vi "Multi-Device_Sync-AI_and_AO-Shared_Timebase_&_Trig-DSA SINGLE DEVICE.vi"() -> ()   [LabVIEW 2020]
doc: "I. Description:\nThis example configures a total of four tasks on two PXI Dynamic Signal Acquistion (DSA) devices. Each device runs a task for analog input and another for analog output. This VI illustrates continuous analog input and ouptut operations.\n\nII. Instructions for Running:\n1. Select which type of Syncrhonization method you want to use.\n2. Select the physical channels to corresponding to the signal connection on each device.\n3. Enter the minimum and maximum expected voltage for the input and output operations on each device.\nNote: For optimal accuracy, match the input range to the expected voltage level of the measured signal (for input) and generated signal (for output).\n4. Set the number of samples to acquire per channel. This parameter determines how many points will be read and generated with each iteration of the WHILE loop.\n5. Set the rate of the acquisition and generation. The same sampling rate is employed for input and output operations on each device.\nNote: The sampling rate should be at least 2.2 times the maximum frequency component of the signal being acquired on analog input and the signal being generated on analog output. Frequency components beyond about 0.47 times the sampling rate will be eliminated by the alias and imaging protection on the DSA device.\n\nIII. Block Diagram Steps:\n1. Create an analog input and output channel for both the master and slave devices.\n2. Set timing parameters for a continuous acquisition. The sample rate and block size are set to the same values for each device.\n3. There are two types of synchronization available on DSA devices. The first method shares the Sample Clock Timebase across the PXI_Star bus. It also uses the Sync Pulse which is shared across the PXI_Trig / RTSI bus. The second method uses the Sync Pulse in conjunction with the PXI Reference clock 10 on the PXI backplane. \n4. Call the Get Terminal Name with Device Prefix VI to append the device name to the signal name for the acquisition start trigger. This signal is then used as an output generation trigger on the master as well as and acquisition start trigger and generation start trigger on the slave. The signal is shared along the PXI_Trig / RTSI bus.\n5. Synthesize a standard waveform (sine, square, or triangle) and load this data into the output RAM buffer for each device.\n6. Call the Start VI to start the acquisition and generation tasks. (Note: The flat case structure provides flow control so that the slave device is armed before the master so that the slave device does not miss the trigger.)\n7. Read all of the waveform data from both devices.\n8. Check the status of the analog output tasks on both devices.\n9. Call the Clear Task VI to stop the acquisition and generation and clear the task.\n10. Use the popup dialog box to display an error if any.\n\nIV. I/O Connections Overview:\nMake sure your signal input and output terminals matches the Physical Channel I/O controls.\n\nIt is important to ensure that your PXI chassis has been properly configured in MAX. If your chassis has not been configured in software before running the VI, your devices may fail to synchronize properly."
uses:
  <vilib>/Utility/error.llb/DialogType.ctl
  <vilib>/DAQmx/write.llb/DAQmx Write (Analog Wfm 1Chan NSamp).vi
  <vilib>/DAQmx/create/channels.llb/DAQmx Create Channel (AI-Voltage-Basic).vi
  <vilib>/DAQmx/create/channels.llb/DAQmx Create Channel (AO-Voltage-Basic).vi
  <vilib>/DAQmx/configure/timing.llb/DAQmx Timing (Sample Clock).vi
  <vilib>/DAQmx/configure/trigger.llb/DAQmx Start Trigger (Digital Edge).vi
  <vilib>/DAQmx/miscellaneous.llb/DAQmx Fill In Error Info.vi
  <vilib>/DAQmx/read.llb/DAQmx Read (Analog 1D Wfm NChan NSamp).vi
  <resource>/objmgr/daqmx.rc
panel:
  out "Resulting Sample \nClock Rate [S/s]":dbl format="%.2f"
  in  "Desired Frequency":dbl=1000.0 format="%.2f"
  in  "Cycles per Buffer":dbl=5.0 format="%.2f"
  in  "Waveform Type":T1(ring)
  in  "Samples per Buffer":dbl=250.0
  in  "Amplitude":dbl=1.0 format="%0.2p"
  in  "Samples per Channel":i32=2000 caption="Samples to Read per Loop"
  in  "Minimum Value":dbl=-10.0 caption="Output Minimum Value" format="%0.2f"
  in  "Maximum Value":dbl=10.0 caption="Output Maximum Value" format="%0.2f"
  in  "Physical Channel":tag="PXI1Slot2/ao0" caption="Master Output Physical Channels"
  in  "Maximum Value":dbl=10.0 caption="Input Maximum Value" format="%0.2f"
  in  "Minimum Value":dbl=-10.0 caption="Input Minimum Value" format="%0.2f"
  in  "Physical Channel":tag="PXI1Slot2/ai0" caption="Master Input Physical Channel"
  in  "stop":bool
  out "Measurement":waveform(dbl)[](graph) caption="Measurement:  Master Board"
  # "For instructions, select Help>>Show Context Help"
  # "Channel Parameters:  Master Board"
  # "Timing Parameters"
  # "Waveform Information"
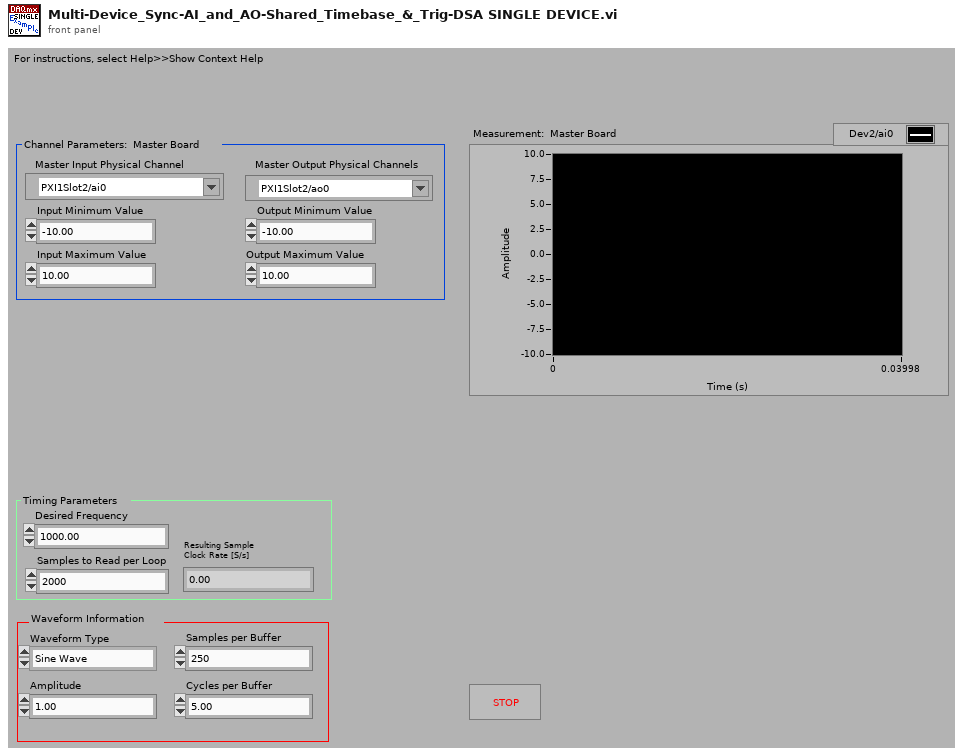
[diagram p1: front panel]
types:
  T1 = enum16{"Sine Wave", "Triangle Wave", "Square Wave", "Sawtooth Wave"}
  T2 = typedef "DialogType.ctl" = u16
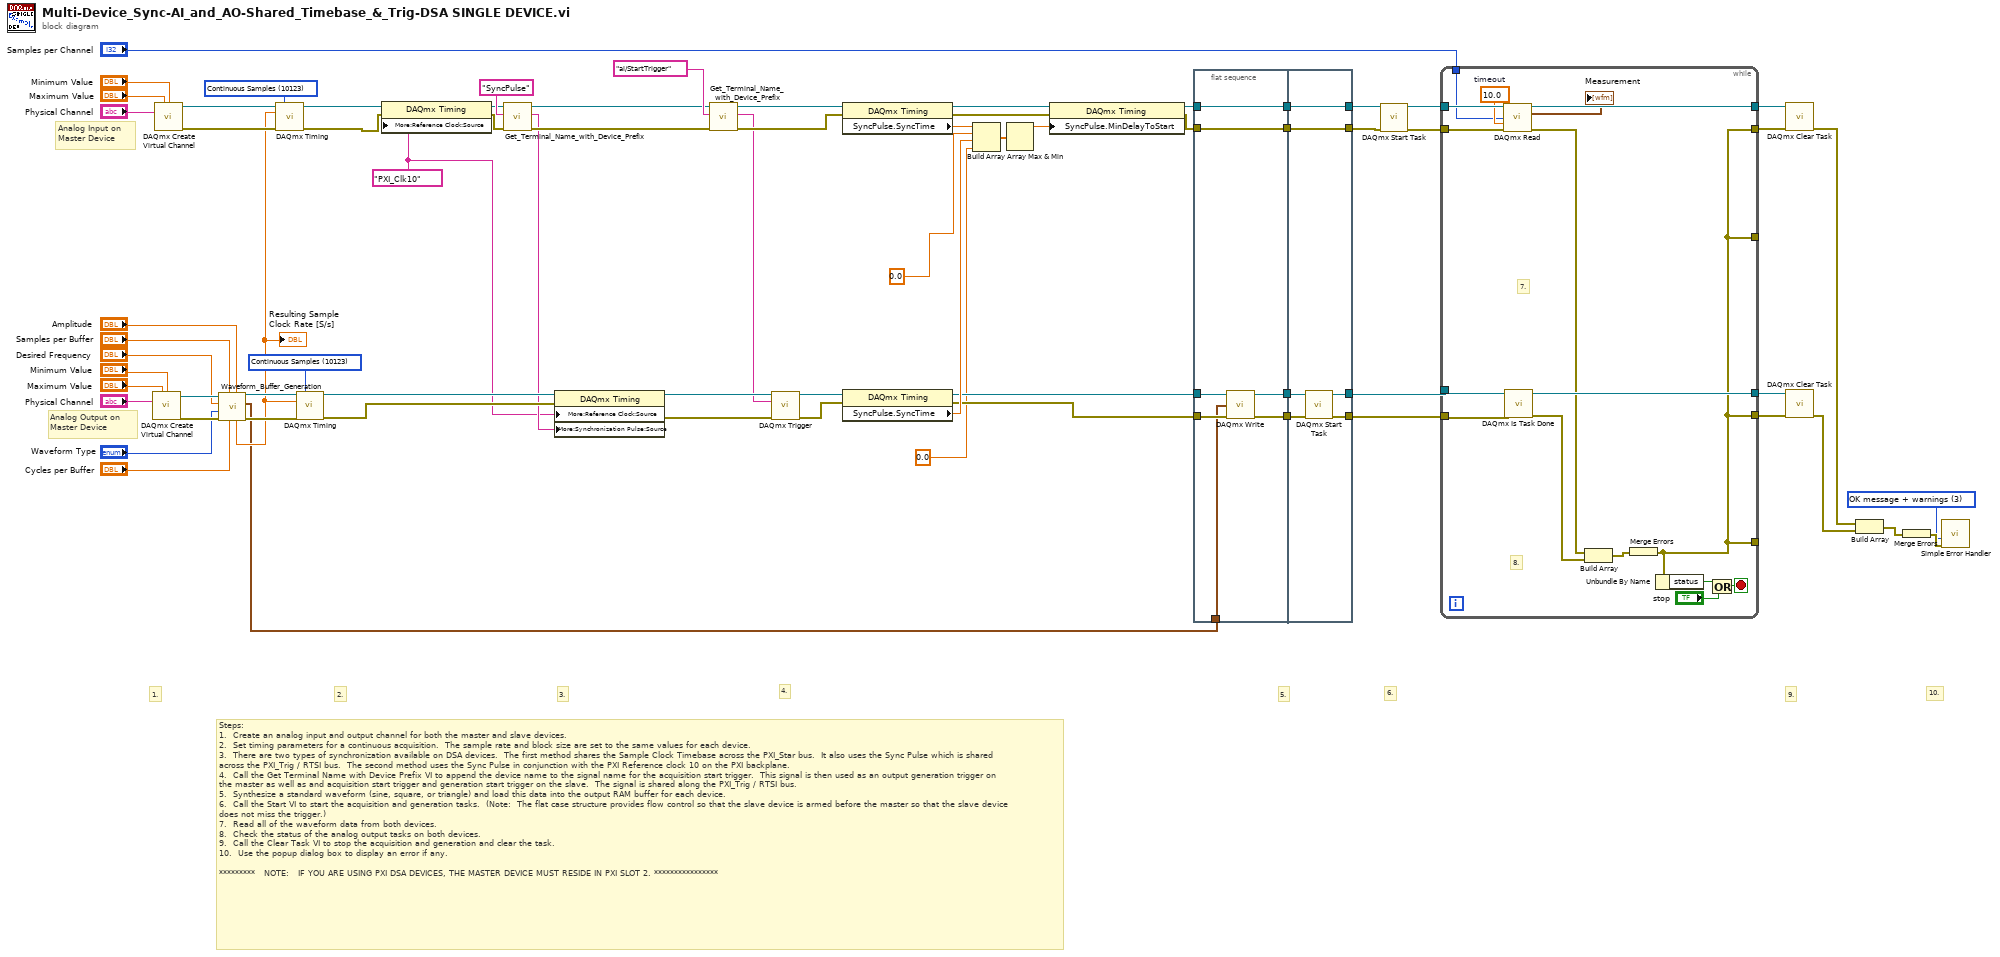
[diagram p0: block diagram]
diagram:
  w3 = tag "PXI_Clk10" ("RefClk.Src")
  w42 = T2 3 items=["no dialog", "OK message", "continue or stop message", "OK message + warnings", "continue/stop + warnings"] ("type of dialog (OK msg:1)")
  w65 = 10123 items=["Finite Samples"=10178, "Continuous Samples"=10123] ("sample mode")
  w68 = 10123 items=["Finite Samples"=10178, "Continuous Samples"=10123] ("sample mode")
  # "Analog Output on\nMaster Device"
  # "Analog Input on\nMaster Device"
  # "10."
  # "9."
  # "Steps: \n1.  Create an analog input and output channel for both the master and slave devices.\n2.  Set timing parameters for a continuous acquisition.  The sample rate and block size are set to the same values for each device.\n3.  There are two types of synchronization available on DSA devices.  The first method shares the Sample Clock Timebase across the PXI_Star bus.  It also uses the Sync Pulse which is shared across the PXI_Trig / RTSI bus.  The second method uses the Sync Pulse in conjunction with the PXI Reference clock 10 on the PXI backplane. \n4.  Call the Get Terminal Name with Device Prefix VI to append the device name to the signal name for the acquisition start trigger.  This signal is then used as an output generation trigger on the master as well as and acquisition start trigger and generation start trigger on the slave.  The signal is shared along the PXI_Trig / RTSI bus.\n5.  Synthesize a standard waveform (sine, square, or triangle) and load this data into the output RAM buffer for each device.\n6.  Call the Start VI to start the acquisition and generation tasks.  (Note:  The flat case structure provides flow control so that the slave device is armed before the master so that the slave device does not miss the trigger.)\n7.  Read all of the waveform data from both devices.\n8.  Check the status of the analog output tasks on both devices.\n9.  Call the Clear Task VI to stop the acquisition and generation and clear the task.\n10.  Use the popup dialog box to display an error if any.\n\n*********   NOTE:  \tIF YOU ARE USING PXI DSA DEVICES, THE MASTER DEVICE MUST RESIDE IN PXI SLOT 2. ****************"
  # "6."
  # "5."
  # "4."
  # "3."
  # "2."
  # "1."
  n1 = call-poly <vilib>:"DAQmx Create Virtual Channel.vi"("maximum value"="Maximum Value", "minimum value"="Minimum Value", "physical channels"="Physical Channel") -> ("task out"=w49:refnum<k21>, "error out"=w48:errorcluster)  [unwired: 11 in]
  n2 = call-poly <vilib>:"DAQmx Create Virtual Channel.vi"("maximum value"="Maximum Value", "minimum value"="Minimum Value", "physical channels"="Physical Channel") -> ("task out"=w70:refnum<k21>, "error out"=w72:errorcluster)  [unwired: 11 in]
  n3 = call "Waveform_Buffer_Generation.vi"("Amplitude"="Amplitude", "Cycles per Buffer"="Cycles per Buffer", "Samples per Buffer"="Samples per Buffer", "error in (no error)"=w48, "Waveform Type"="Waveform Type", "Desired Frequency"="Desired Frequency", "task/channels in"=w49) -> ("error out"=w47:errorcluster, "Waveform"=w9:waveform(dbl), "task out"=w50:refnum<k21>, "Resulting Sample Clock Rate"=w33:dbl)  [unwired: 1 out]
  "Resulting Sample \nClock Rate [S/s]" <- w33
  n4 = call-poly <vilib>:"DAQmx Timing.vi"("task/channels in"=w70, "sample mode"=w68, "rate"=w33, "error in"=w72) -> ("task out"=w67:refnum<k21>, "error out"=w66:errorcluster)  [unwired: 10 in]
  n5 = call-poly <vilib>:"DAQmx Timing.vi"("task/channels in"=w50, "sample mode"=w65, "rate"=w33, "error in"=w47) -> ("task out"=w41:refnum<k21>, "error out"=w40:errorcluster)  [unwired: 10 in]
  n6 = property class="DAQmx Timing"(reference=w67, error in=w66, "More:Reference Clock:Source"=w3) -> (reference out=w4:refnum<k21>, error out=w2:errorcluster)
  n7 = call "Get_Terminal_Name_with_Device_Prefix.vi"("error in (no error)"=w2, "Local Terminal Name"="SyncPulse", "task/channels in"=w4) -> ("error out"=w28:errorcluster, "Terminal Name with Device Prefix"=w5:tag, "task out"=w29:refnum<k21>)  [unwired: 6 in]
  n8 = property class="DAQmx Timing"(reference=w41, error in=w40, "More:Reference Clock:Source"=w3, "More:Synchronization Pulse:Source"=w5) -> (reference out=w32:refnum<k21>, error out=w31:errorcluster)
  n9 = call "Get_Terminal_Name_with_Device_Prefix.vi"("error in (no error)"=w28, "Local Terminal Name"="ai/StartTrigger", "task/channels in"=w29) -> ("error out"=w26:errorcluster, "Terminal Name with Device Prefix"=w1:tag, "task out"=w27:refnum<k21>)  [unwired: 6 in]
  n10 = call-poly <vilib>:"DAQmx Trigger.vi"("task/channels in"=w32, "source"=w1, "error in"=w31) -> ("task out"=w24:refnum<k21>, "error out"=w25:errorcluster)  [unwired: 11 in]
  n11 = property class="DAQmx Timing"(reference=w27, error in=w26) -> (reference out=w21:refnum<k21>, error out=w22:errorcluster, "SyncPulse.SyncTime"=w23:dbl)
  n12 = property class="DAQmx Timing"(reference=w24, error in=w25) -> (reference out=w12:refnum<k21>, error out=w13:errorcluster, "SyncPulse.SyncTime"=w18:dbl)
  n13 = Build Array(w23, 0.0, w18, 0.0) -> (w20:dbl[])
  n14 = Array Max & Min(array=w20) -> (max value=w19:dbl)  [unwired: 3 out]
  n15 = property class="DAQmx Timing"(reference=w21, error in=w22, "SyncPulse.MinDelayToStart"=w19) -> (reference out=w16:refnum<k21>, error out=w17:errorcluster)
  n16 = flat-sequence {
    tunnel: [w79] -> w15
    tunnel: [w78] -> w14
    tunnel: [w75] -> w11
    tunnel: [w74] -> w10
    tunnel: w9 -> [w73]
    tunnel: w16 -> [w79]
    tunnel: w17 -> [w78]
    tunnel: w13 -> [w77]
    tunnel: w12 -> [w76]
    tunnel: [w84] -> w51
    tunnel: [w85] -> w52
    tunnel: [w83] -> w39
    tunnel: [w82] -> w37
    tunnel: w15 -> [w83]
    tunnel: w14 -> [w82]
    tunnel: w11 -> [w81]
    tunnel: w10 -> [w80]
    frame #0 {
      n17 = call-poly <vilib>:"DAQmx Write.vi"("task/channels in"=w76, "data"=w73, "error in"=w77) -> ("task out"=w74:refnum<k21>, "error out"=w75:errorcluster)  [unwired: 10 in, 1 out]
    }
    frame #1 {
      n18 = call <vilib>:"DAQmx Start Task.vi"("task/channels in"=w80, "error in"=w81) -> ("task out"=w85:refnum<k21>, "error out"=w84:errorcluster)  [unwired: 12 in]
    }
  }
  n19 = call <vilib>:"DAQmx Start Task.vi"("task/channels in"=w39, "error in"=w37) -> ("task out"=w38:refnum<k21>, "error out"=w36:errorcluster)  [unwired: 12 in]
  n20 = while {
    tunnel: [w90] -> w71
    tunnel: w38 -> [w101]
    tunnel: [w100] -> w69
    tunnel: [w90] -> _
    tunnel: w52 -> [w98]
    tunnel: w36 -> [w92]
    tunnel: [w97] -> w64
    tunnel: [w90] -> w63
    tunnel: [w90] -> _
    tunnel: w51 -> [w91]
    tunnel: "Samples per Channel" -> [w89]
    stop <- w94 stop-if-true
    w99 = 10.0  # timeout
    # "8."
    # "7."
    n21 = call-poly <vilib>:"DAQmx Read.vi"("task/channels in"=w101, "number of samples per channel"=w89, "timeout"=w99, "error in"=w92) -> ("task out"=w100:refnum<k21>, "data"=→"Measurement":waveform(dbl)[], "error out"=w87:errorcluster)  [unwired: 9 in]
    n22 = call <vilib>:"DAQmx Is Task Done.vi"("task/channels in"=w98, "error in"=w91) -> ("task out"=w97:refnum<k21>, "error out"=w88:errorcluster)  [unwired: 11 in, 1 out]
    n23 = Build Array(w87, w88) -> (w96:errorcluster[])
    n24 = Merge Errors(w96) -> (w90:errorcluster)
    n25 = Unbundle By Name(w90) -> ("status"=w95:bool)
    n26 = Or(x=w95, y="stop") -> (x .or. y?=w94:bool)
  }
  n27 = call <vilib>:"DAQmx Clear Task.vi"("task in"=w69, "error in"=w71) -> ("error out"=w62:errorcluster)  [unwired: 13 in]
  n28 = call <vilib>:"DAQmx Clear Task.vi"("task in"=w64, "error in"=w63) -> ("error out"=w61:errorcluster)  [unwired: 13 in]
  n29 = Build Array(w62, w61) -> (w60:errorcluster[])
  n30 = Merge Errors(w60) -> (w59:errorcluster)
  n31 = call <vilib>:"Simple Error Handler.vi"("type of dialog (OK msg:1)"=w42, "error in (no error)"=w59) -> ()  [unwired: 3 in, 5 out]
